vi "IMAQ balance energy.vi"(10 "Target Image":T1, 11 "Base Image":T1) -> (3 "Normalized Target":T1(plugin-control))   [LabVIEW 2012, in "LightPipes.lvlib"]
uses:
  LightPipes.lvlib
  <vilib>/vision/Image Controls.llb/IMAQ Image.ctl
panel:
  out "Target":i32
  out "Base":i32
  out "Normalized":i32
  # "1. Normalize Target.\n\n2. Scale Target's energy to Base's."
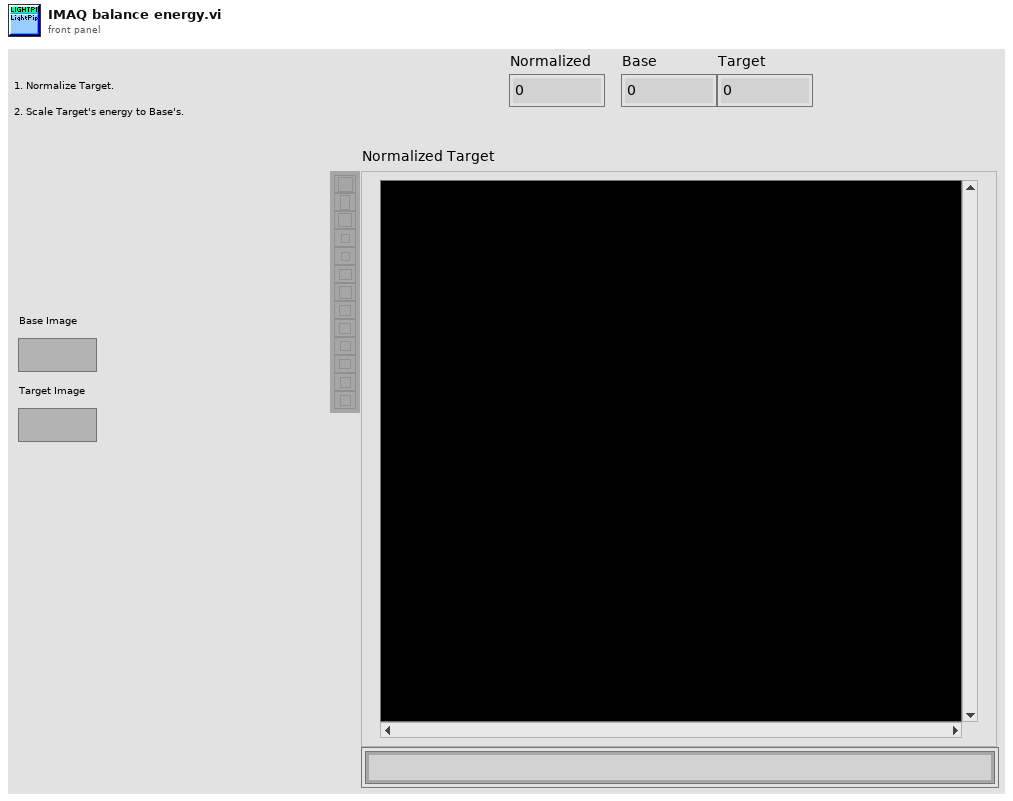
[diagram p1: front panel]
types:
  T1 = typedef "IMAQ Image.ctl" = refnum<image>
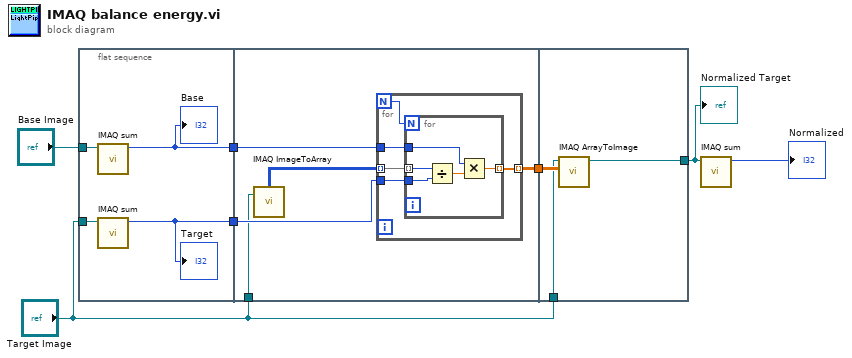
[diagram p0: block diagram]
diagram:
  n1 = flat-sequence {
    tunnel: [w11] -> w6
    tunnel: [w10] -> w5
    tunnel: "Base Image" -> [w9]
    tunnel: "Target Image" -> [w8]
    tunnel: w6 -> [w15]
    tunnel: w5 -> [w14]
    tunnel: [w13] -> w4
    tunnel: "Target Image" -> [w12]
    tunnel: w4 -> [w29]
    tunnel: "Target Image" -> [w28]
    tunnel: [w27] -> w1
    frame #0 {
      n2 = call "IMAQ sum.vi"("Image"=w9) -> ("Sum"=w10:i32)  [unwired: 10 in]
      "Base" <- w10
      n3 = call "IMAQ sum.vi"("Image"=w8) -> ("Sum"=w11:i32)  [unwired: 10 in]
      "Target" <- w11
    }
    frame #1 {
      n4 = call "IMAQ ImageToArray"("Image"=w12) -> ("Image Pixels (U8)"=w16:u8[][])  [unwired: 3 in, 4 out]
      n5 = for {
        N -> [w21]
        tunnel: w16 -> [w20] mode=indexing
        tunnel: [w19] -> w13 mode=indexing
        tunnel: w15 -> [w18]
        tunnel: w14 -> [w17]
        n6 = for {
          N: w21 -> [_]
          tunnel: w20 -> [w26] mode=indexing
          tunnel: [w24] -> w19 mode=indexing
          tunnel: w18 -> [w23]
          tunnel: w17 -> [w22]
          n7 = Divide(x=w26, y=w23) -> (x/y=w25:dbl)
          n8 = Multiply(x=w22, y=w25) -> (x*y=w24:dbl)
        }
      }
    }
    frame #2 {
      n9 = call "IMAQ ArrayToImage"("Image Pixels (U8)"=w29, "Image"=w28) -> ("Image Out"=w27:T1)  [unwired: 8 in, 1 out]
    }
  }
  n10 = call "IMAQ sum.vi"("Image"=w1) -> ("Sum"=→"Normalized":i32)  [unwired: 10 in]
  "Normalized Target" <- w1
